vi "3_VI_XL-MaxSonar.vi"(0 "Analog IN [V]":dbl) -> (7 "Sonar Distance":dbl)   [LabVIEW 2019]
panel:
  in  "Offset":dbl=5.0
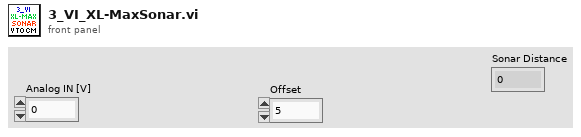
[diagram p1: front panel]
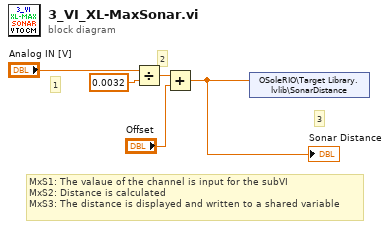
[diagram p0: block diagram]
diagram:
  # "3"
  # "2"
  # "1"
  # "MxS1: The valaue of the channel is input for the subVI\nMxS2: Distance is calculated\nMxS3: The distance is displayed and written to a shared variable"
  n1 = Divide(x="Analog IN [V]", y=0.0032) -> (x/y=w4:dbl)
  n2 = Add(x=w4, y="Offset") -> (x+y=w1:dbl)
  "Sonar Distance" <- w1
  n3 = shared-variable "OSoleRIO\\Target Library.lvlib\\SonarDistance"(w1) -> ()  [unwired: 1 in, 1 out]
